vi "Write DomeCommunicator.vi"(8 "error in (no error)":errorcluster, 10 "DomeCommunicator.lvclass":refnum<class "DomeCommunicator.lvclass">, 11 "DomeController in":refnum<class "DomeController.lvclass">) -> (0 "error out":errorcluster, 3 "DomeController out":refnum<class "DomeController.lvclass">)   [LabVIEW 2016, in "DomeController.lvclass"]
uses:
  DomeController.lvclass
  domeCommunicator/DomeCommunicator.lvclass
  DomeController.lvclass/DomeController.ctl
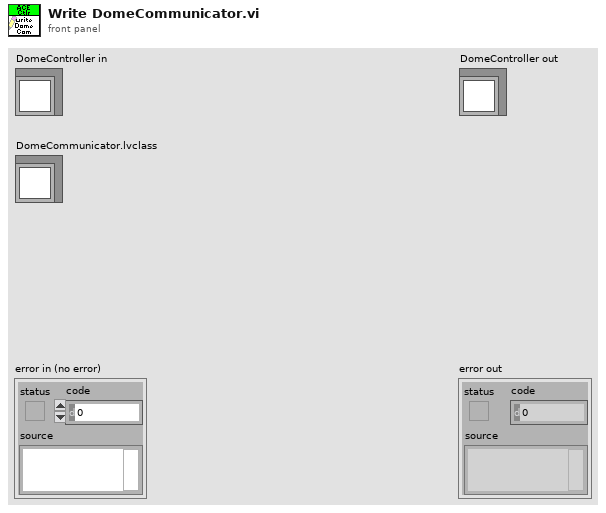
[diagram p1: front panel]
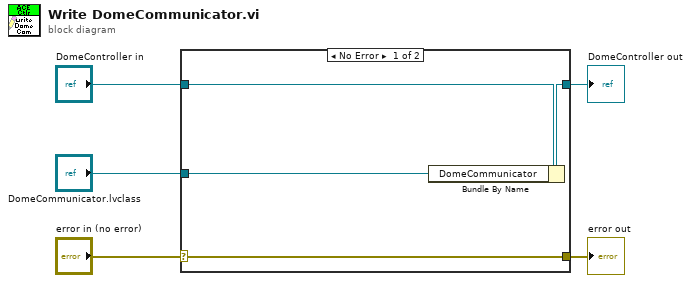
[diagram p0: block diagram]
diagram:
  n1 = case shown="No Error" "error in (no error)" {
    selector: "error in (no error)" -> [w9 w10]
    tunnel: [w9 w10] -> w4
    tunnel: [w7 w11] -> w2
    tunnel: "DomeController in" -> [w8 w11]
    tunnel: "DomeCommunicator.lvclass" -> [w6 _]
    frame No Error {
      n2 = Bundle By Name(cluster=w8, "DomeCommunicator"=w6) -> (w7:refnum<class "DomeController.lvclass">)
    }
    frame Error {
    }
  }
  "error out" <- w4
  "DomeController out" <- w2
